vi "Set Color.vi"(8 "error in (no error)":errorcluster, 10 "Color Message.lvclass":refnum<class "Color Message.lvclass">, 11 "[V] Main UI in":refnum<class "[V] Main UI.lvclass">) -> (0 "error out":errorcluster, 3 "[V] Main UI out":refnum<class "[V] Main UI.lvclass">)   [LabVIEW 2020, in "[V] Main UI.lvlib" / "[V] Main UI.lvclass"]
uses:
  [V] Main UI.lvclass
  Color Interface/Color/Color Message.lvclass
  Color Interface/Color/Color Message.lvclass/Color Message.ctl
  Depden On/Abstruct View/Abstruct View/Abstruct View.lvclass/Abstruct View.ctl
  Depden On/Abstruct View/Abstruct View/Data Accessors/Read Core VI.vi
  Color Interface/Color/Accessors/Read BG Color.vi
  Color Interface/Color/Accessors/Read Fornt Color.vi
  Color Interface/Color/Accessors/Read txt Color.vi
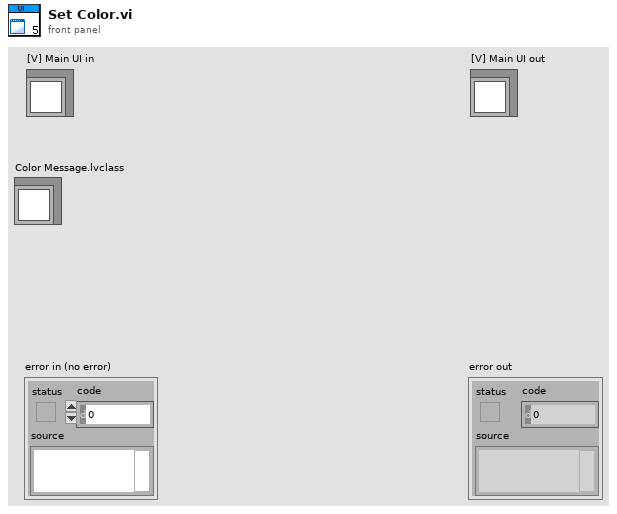
[diagram p1: front panel]
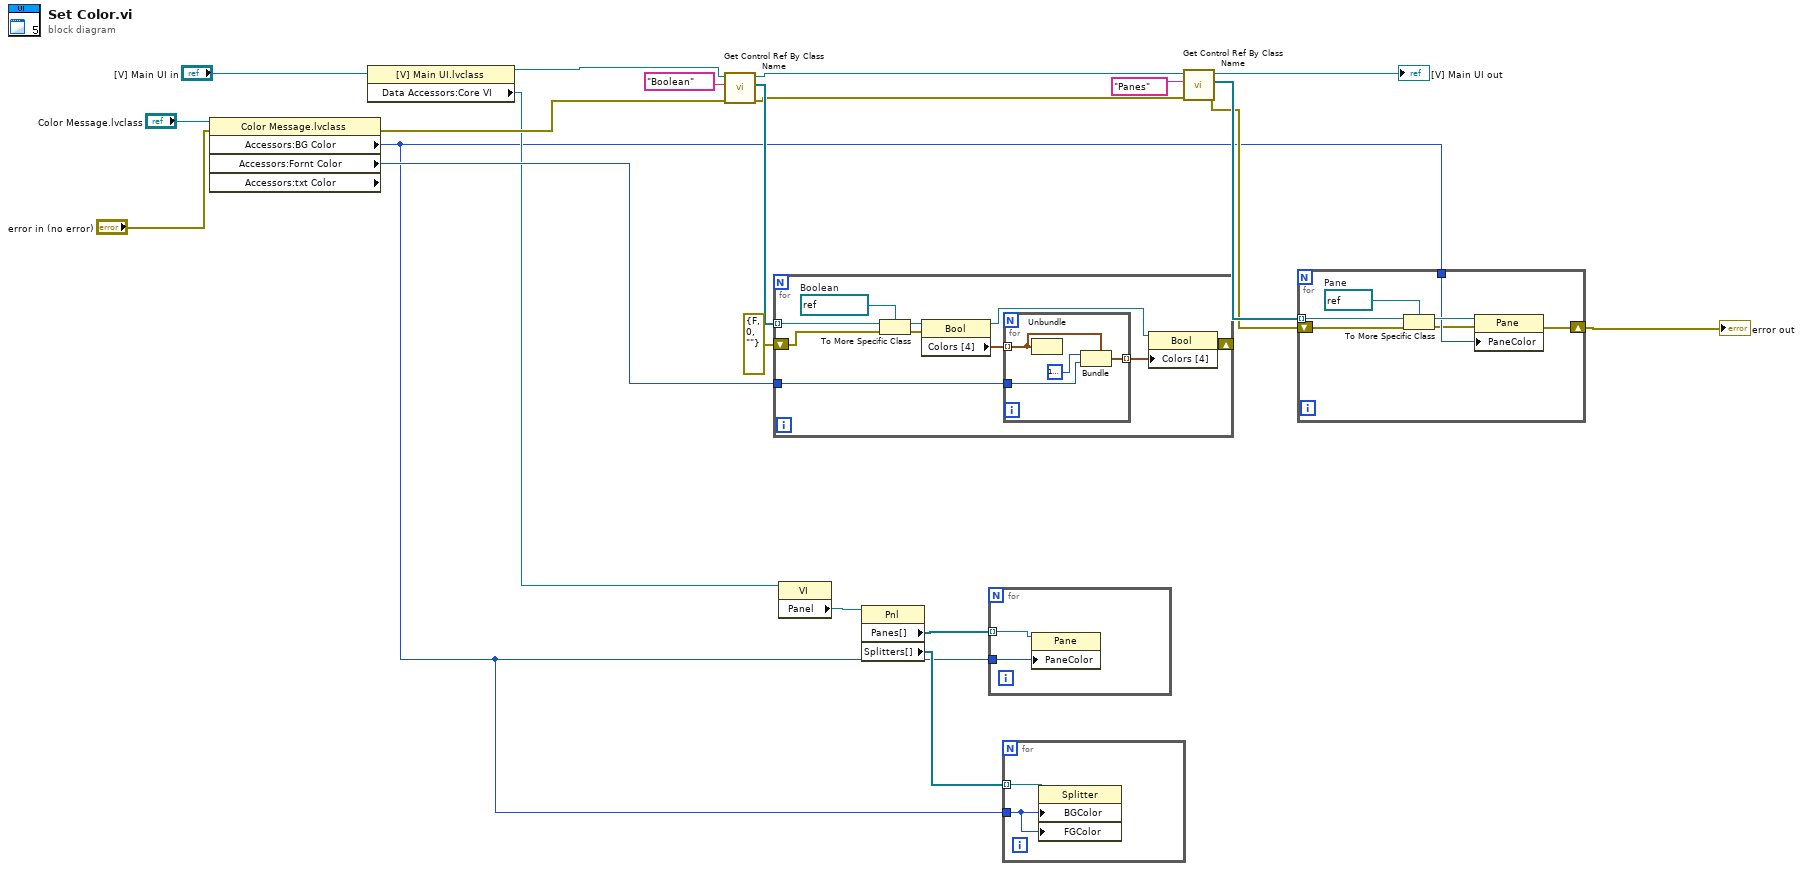
[diagram p0: block diagram]
diagram:
  n1 = property class="Color Message.lvclass" props=["Accessors:BG Color", "Accessors:Fornt Color", "Accessors:txt Color"](reference="Color Message.lvclass", error in="error in (no error)") -> (error out=w17:errorcluster, "Accessors:BG Color"=w1:u32, "Accessors:Fornt Color"=w18:u32)  [unwired: 2 out]
  n2 = property class="[V] Main UI.lvclass"(reference="[V] Main UI in") -> (reference out=w5:refnum<class "[V] Main UI.lvclass">, "Data Accessors:Core VI"=w4:refnum<vi>)  [unwired: 1 in, 1 out]
  n3 = call "Get Control Ref By Class Name.vi"("error in (no error)"=w17, "Control Class"="Boolean", "[V] Main UI in"=w5) -> ("error out"=w15:errorcluster, "refs"=w19:refnum<vi>[], "[V] Main UI out"=w16:refnum<class "[V] Main UI.lvclass">)  [unwired: 6 in]
  n4 = for {
    tunnel: w19 -> [w31] mode=indexing
    tunnel: w18 -> [w25]
    shift-right: [w24] -> _
    shift-left: errorcluster {"status"=FALSE, "code"=0, "source"=""} ("error out") -> [w23]
    w30 = refnum<vi> refnum  # Boolean
    n5 = To More Specific Class(target class=w30, reference=w31, error in=w23) -> (specific class reference=w29:refnum<vi>, error out=w22:errorcluster)
    n6 = property class="Bool"(reference=w29, error in=w22) -> (reference out=w27:refnum<vi>, "Colors [4]"=w28:cluster{u32, u32}[])  [unwired: 1 out]
    n7 = for {
      tunnel: w28 -> [w34] mode=indexing
      tunnel: [w35] -> w26 mode=indexing
      tunnel: w25 -> [w33]
      n8 = Unbundle(w34) -> ()  [unwired: 2 out]
      n9 = Bundle(cluster=w34, u32 16777216, w33) -> (w35:cluster{u32, u32})
    }
    n10 = property class="Bool"(reference=w27, "Colors [4]"=w26) -> (error out=w24:errorcluster)  [unwired: 1 in, 1 out]
  }
  n11 = property class="VI"(reference=w4) -> ("Panel"=w7:refnum<vi>)  [unwired: 1 in, 2 out]
  n12 = property class="Pnl"(reference=w7) -> ("Panes[]"=w3:refnum<vi>[], "Splitters[]"=w2:refnum<vi>[])  [unwired: 1 in, 2 out]
  n13 = for {
    tunnel: w3 -> [w37] mode=indexing
    tunnel: w1 -> [w36]
    n14 = property class="Pane"(reference=w37, "PaneColor"=w36) -> ()  [unwired: 1 in, 2 out]
  }
  n15 = for {
    tunnel: w2 -> [w39] mode=indexing
    tunnel: w1 -> [w38]
    n16 = property class="Splitter"(reference=w39, "BGColor"=w38, "FGColor"=w38) -> ()  [unwired: 1 in, 2 out]
  }
  n17 = call "Get Control Ref By Class Name.vi"("error in (no error)"=w15, "Control Class"="Panes", "[V] Main UI in"=w16) -> ("error out"=w8:errorcluster, "refs"=w12:refnum<vi>[], "[V] Main UI out"=→"[V] Main UI out":refnum<class "[V] Main UI.lvclass">)  [unwired: 6 in]
  n18 = for {
    tunnel: w12 -> [w46] mode=indexing
    tunnel: w1 -> [w43]
    shift-right: [w41] -> w10
    shift-left: w8 -> [w40]
    w45 = refnum<vi> refnum  # Pane
    n19 = To More Specific Class(target class=w45, reference=w46, error in=w40) -> (specific class reference=w44:refnum<vi>, error out=w42:errorcluster)
    n20 = property class="Pane"(reference=w44, error in=w42, "PaneColor"=w43) -> (error out=w41:errorcluster)  [unwired: 1 out]
  }
  "error out" <- w10
